vi "Serial_Transmision_Send_Only.vi"(8 "Command":u8=1 min=1 max=1, 9 "Array":u16[](array[numeric]), 10 "error in":errorcluster, 11 "VISA Refnum in":refnum<visa-resource-name>="COM1") -> (2 "askii Characters":string, 4 "error?":bool, 5 "Transmision uint8 array":u8[](array[numeric]), 6 "Transmision Data in Hex":u8[](array[numeric]) format="%x", 7 "return count":u32)   [LabVIEW 2012]
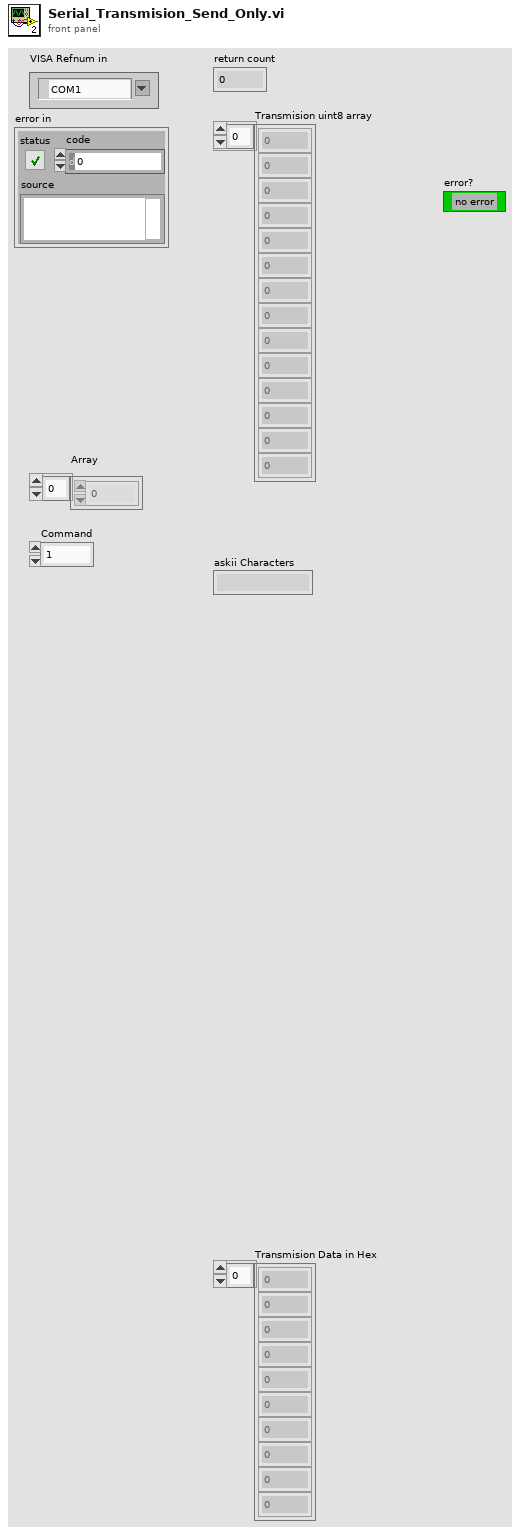
[diagram p1: front panel]
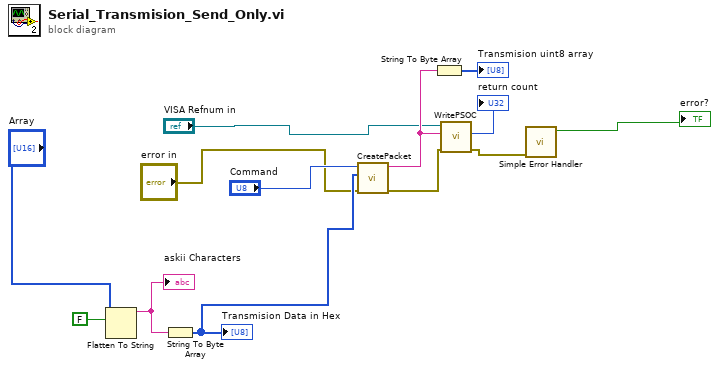
[diagram p0: block diagram]
diagram:
  n1 = Flatten To String(anything="Array", prepend array or string size? (T)=FALSE) -> (data string=w10:string)  [unwired: 2 in, 2 out]
  "askii Characters" <- w10
  n2 = String To Byte Array(string=w10) -> (unsigned byte array=w12:u8[])
  "Transmision Data in Hex" <- w12
  n3 = call "CreatePacket.vi"("error in"="error in", "data"=w12, "command"="Command") -> ("error out"=w5:errorcluster, "Command String"=w7:string)  [unwired: 6 in, 1 out]
  n4 = String To Byte Array(string=w7) -> (unsigned byte array=→"Transmision uint8 array":u8[])
  n5 = call "WritePSOC.vi"("error in"=w5, "write buffer"=w7, "VISA resource name"="VISA Refnum in") -> ("error out"=w3:errorcluster, "return count"=→"return count":u32)  [unwired: 5 in, 1 out]
  n6 = call <vilib>:"Simple Error Handler.vi"("error in (no error)"=w3) -> ("error?"=→"error?":bool)  [unwired: 4 in, 4 out]
